vi "test_Create Global MetaData Channel_error on name collision.vi"(8 "error in (no error)":errorcluster, 11 "TestCase in":refnum<class "Instrument Addon Scripting API Channels Unit Tests.lvclass">) -> (0 "error out":errorcluster, 3 "TestCase out":refnum<class "Instrument Addon Scripting API Channels Unit Tests.lvclass">)   [LabVIEW 2019, in "Instrument Addon Scripting API Channels Unit Tests.lvclass"]
uses:
  Instrument Addon Scripting API Channels Unit Tests.lvclass
  APIs/Scripting API/TypeDefs/Array Type Cast Settings.ctl
  APIs/Scripting API/TypeDefs/Array Element.ctl
  Addon/Addon Shared/Types/Type Cast Type.ctl
  Addon/Addon Shared/Types/Endian.ctl
  Instrument Addon Scripting API Channels Unit Tests.lvclass/Instrument Addon Scripting API Channels Unit Tests.ctl
  APIs/Scripting API/Channels/Create Global MetaData Channel - Array - Type Cast.vi
  <vilib>/addons/_JKI Toolkits/VI Tester/TestCase.llb/TestCase.lvclass
  Instrument Addon Scripting API Test Assets/Instrument Addon Scripting API Test Assets.lvclass
  APIs/Scripting API/Instrument Addon Scripting API.lvlib
  Addon/Addon Shared/Instrument Addon Shared.lvlib
  C:/Program Files (x86)/National Instruments/LabVIEW 2019/vi.lib/addons/_JKI Toolkits/VI Tester/TestCase.llb/TestCase.lvclass
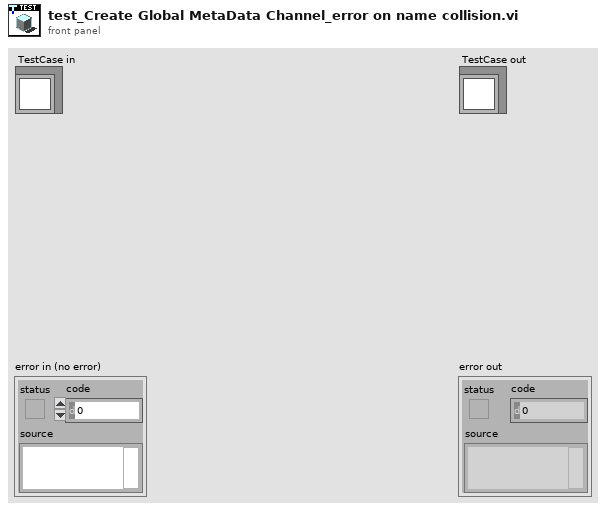
[diagram p1: front panel]
types:
  T1 = typedef "Instrument Addon Scripting API.lvlib/Array Type Cast Settings.ctl" = cluster{"Elements":T2[], "Delimiter":string, "Type":T3, "Endian":T4}
  T2 = typedef "Instrument Addon Scripting API.lvlib/Array Element.ctl" = cluster{"Name":string, "Default Value":dbl, "Units":string}
  T3 = typedef "Instrument Addon Shared.lvlib/Type Cast Type.ctl" = enum16{"DBL", "SGL", "U64", "U32", "U16", "U8", "I64", "I32", "I16", "I8"}
  T4 = typedef "Instrument Addon Shared.lvlib/Endian.ctl" = enum16{"Native", "Little", "Big"}
  T5 = typedef "Custom Device API.lvlib/Custom Device Item Ref.ctl" = u64
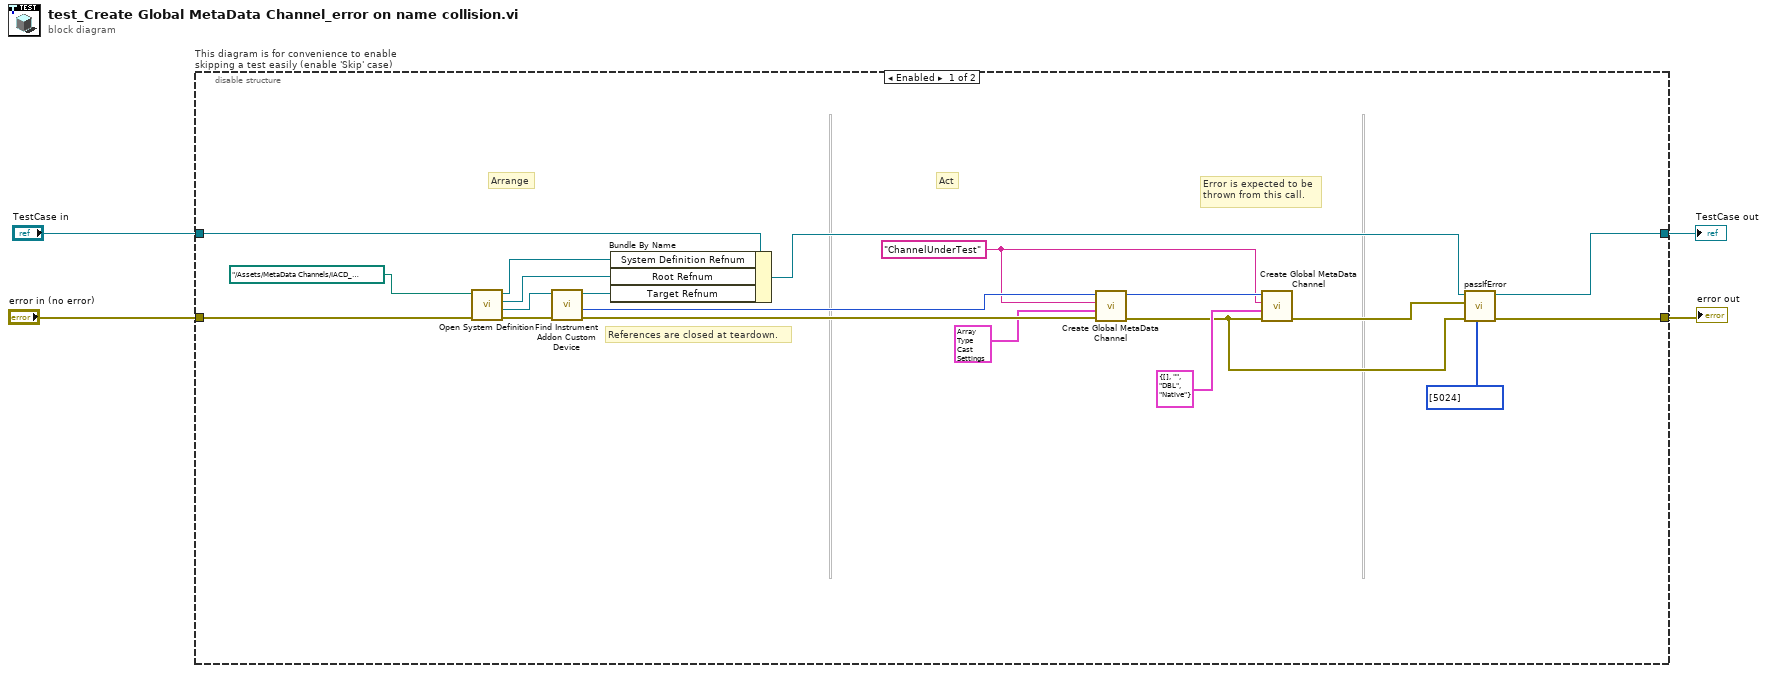
[diagram p0: block diagram]
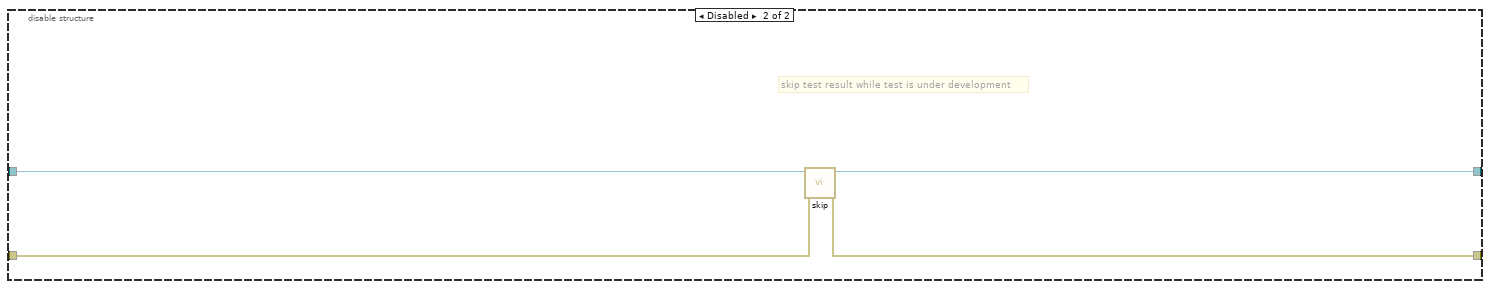
[diagram p2: hidden frame]
diagram:
  n1 = disable-structure "This diagram is for convenience to enable skipping a test easily (enable 'Skip' case)" shown="Enabled" {
    disable-tunnel: "TestCase in" -> [w18 w28]
    disable-tunnel: [w15 w26] -> w1
    disable-tunnel: [w14 w27] -> w3
    disable-tunnel: "error in (no error)" -> [w24 w25]
    frame Enabled {
      w11 = "ChannelUnderTest" ("Name")
      # "Error is expected to be\nthrown from this call."
      # "References are closed at teardown."
      # "Act"
      # "Arrange"
      n2 = call "Open System Definition.vi"("error in (no error)"=w24, "System Definition File"=path "../Assets/MetaData Channels/IACD_channels.nivssdf") -> ("error out"=w22:errorcluster, "Target Refnum"=w23:refnum<k24>, "Root Refnum"=w20:refnum<k24>, "System Definition Refnum"=w19:refnum<k24>)  [unwired: 6 in]
      n3 = call "Find Instrument Addon Custom Device.vi"("error in"=w22, "target in"=w23) -> ("error out"=w16:errorcluster, "NodeID"=w17:u64, "target out"=w21:refnum<k24>)  [unwired: 7 in]
      n4 = Bundle By Name(cluster=w18, "System Definition Refnum"=w19, "Root Refnum"=w20, "Target Refnum"=w21) -> (w9:refnum<class "Instrument Addon Scripting API Channels Unit Tests.lvclass">)
      n5 = call-poly "Create Global MetaData Channel.vi"("error in (no error)"=w16, "settings"=T1 {"Elements"=[{"Name"="foo", "Default Value"=8.0, "Units"=""}, {"Name"="bar", "Default Value"=9.0, "Units"=""}, {"Name"="baz", "Default Value"=10.0, "Units"="h"}], "Delimiter"="-", "Type"=enum."I8", "Endian"=enum."Native"} ("Settings"), "channel name"=w11, "instrument addon refnum in"=w17) -> ("error out"=w6:errorcluster, "instrument addon refnum out"=w12:T5)  [unwired: 4 in, 2 out]
      n6 = call-poly "Create Global MetaData Channel.vi"("error in (no error)"=w6, "settings"=T1 {"Elements"=[], "Delimiter"="", "Type"=enum."DBL", "Endian"=enum."Native"} ("Settings"), "channel name"=w11, "instrument addon refnum in"=w12) -> ("error out"=w7:errorcluster)  [unwired: 4 in, 3 out]
      n7 = call-dynamic "passIfError.vi"("passing error codes (default = any error code)"=i32[] [5024], "error in (no error)"=w6, "error"=w7, "TestCase in"=w9) -> ("error out"=w14:errorcluster, "TestCase out"=w15:refnum<class "Instrument Addon Scripting API Channels Unit Tests.lvclass">)  [unwired: 6 in]
    }
    frame Disabled {
      # "skip test result while test is under development"
      n8 = call <vilib>:"skip.vi"("error in (no error)"=w25, "TestCase in"=w28) -> ("error out"=w27:errorcluster, "TestCase out"=w26:refnum<class "Instrument Addon Scripting API Channels Unit Tests.lvclass">)  [unwired: 8 in]
    }
  }
  "error out" <- w3
  "TestCase out" <- w1
